vi "Set Function A.vi"(9 "function A (z/y:0)":i16(slide)=1 scale=0.0..3.0, 11 "GPIB addess":string="17") -> ()   [LabVIEW 2017, in "HP4192A IA.lvclass"]
uses:
  HP4192A IA.lvclass
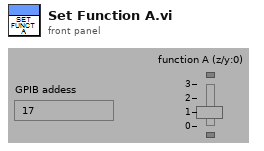
[diagram p1: front panel]
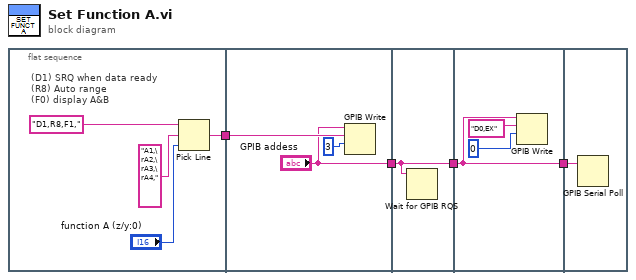
[diagram p0: block diagram]
diagram:
  n1 = flat-sequence {
    tunnel: [w5] -> w4
    tunnel: w4 -> [w10]
    tunnel: ["GPIB addess"] -> w3
    tunnel: w3 -> [w12]
    tunnel: [w12] -> w2
    tunnel: w2 -> [w13]
    tunnel: [w13] -> w1
    tunnel: w1 -> [w16]
    frame #0 {
      # "(D1) SRQ when data ready\n(R8) Auto range\n(F0) display A&B"
      n2 = Pick Line(string ("")="D1,R8,F1,", multi-line string="A1,\rA2,\rA3,\rA4,", line index="function A (z/y:0)") -> (output string=w5:string)
    }
    frame #1 {
      n3 = GPIB Write(0:"GPIB addess", 1:w10, 2:3) -> ()  [unwired: 2 in, 2 out]
    }
    frame #2 {
      n4 = Wait for GPIB RQS(4:w12) -> ()  [unwired: 2 in, 2 out]
    }
    frame #3 {
      n5 = GPIB Write(0:w13, 1:"D0,EX", 2:0) -> ()  [unwired: 2 in, 2 out]
    }
    frame #4 {
      n6 = GPIB Serial Poll(0:w16) -> ()  [unwired: 1 in, 3 out]
    }
  }
